vi "Get Trace State.vi"(4 "Error In":errorcluster, 7 "Trace Point Index":i32) -> (0 "Error Out":errorcluster, 3 "Trace Point State":enum16{"Disabled", "Enabled"}(ring))   [LabVIEW 2014, in "Debugging.lvlib"]
uses:
  Debugging.lvlib
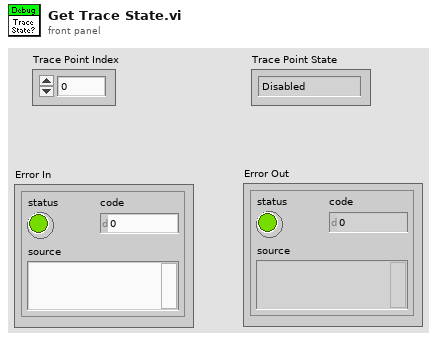
[diagram p1: front panel]
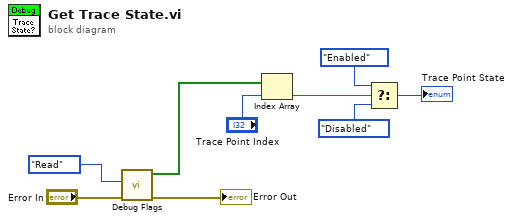
[diagram p0: block diagram]
diagram:
  n1 = call "Debug Flags.vi"("Error In"="Error In", "Function"=enum16{"Read", "Write"}."Read") -> ("Error Out"=→"Error Out":errorcluster, "Trace Flags Out"=w6:bool[])  [unwired: 4 in]
  n2 = Index Array(array=w6, index="Trace Point Index") -> (element=w4:bool)
  n3 = Select(t=enum16{"Disabled", "Enabled"}."Enabled" ("Trace Point State"), s=w4, f=enum16{"Disabled", "Enabled"}."Disabled" ("Trace Point State")) -> (s? t:f=→"Trace Point State":enum16{"Disabled", "Enabled"})
